vi "testGetDataTypeEvent.vi"(8 "error in (no error)":errorcluster) -> (0 "error out":errorcluster)   [LabVIEW 2018]
uses:
  src/LibReader/LibReader.lvclass
  <vilib>/addons/_JKI Toolkits/Caraya/classes/Assert/Assert Error.vi
  <vilib>/addons/_JKI Toolkits/Caraya/classes/Assert/Assert Equal Value_Variant.vi
  <vilib>/addons/_JKI Toolkits/Caraya/classes/Test/Test.lvclass
  <vilib>/addons/_JKI Toolkits/Caraya/classes/Assert/Assert.lvclass
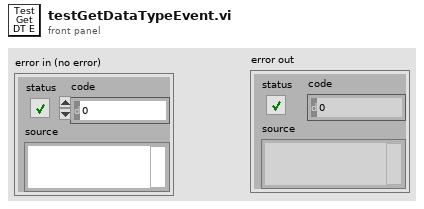
[diagram p1: front panel]
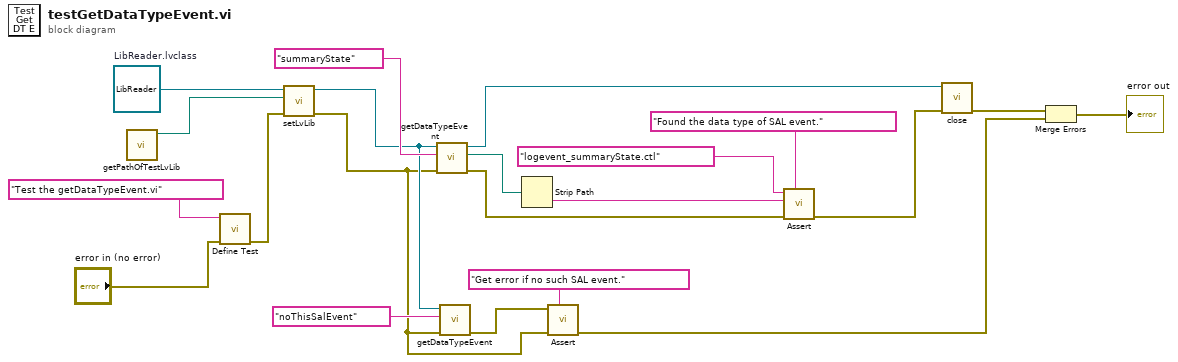
[diagram p0: block diagram]
diagram:
  w19 = refnum<class "LibReader.lvclass"> refnum  # LibReader.lvclass
  n1 = call "getPathOfTestLvLib.vi"() -> ("testLvLibPath"=w18:path)  [unwired: 11 in]
  n2 = call <vilib>:"Define Test.vi"("error in (no error)"="error in (no error)", "Label (VI Title)"="Test the getDataTypeEvent.vi") -> ("error out"=w17:errorcluster)  [unwired: 9 in]
  n3 = call "setLvLib.vi"("error in (no error)"=w17, "pathLvLib"=w18, "LibReader in"=w19) -> ("error out"=w1:errorcluster, "LibReader out"=w8:refnum<class "LibReader.lvclass">)  [unwired: 7 in]
  n4 = call "getDataTypeEvent.vi"("error in (no error)"=w1, "name"="summaryState", "LibReader in"=w8) -> ("error out"=w13:errorcluster, "pathDataType"=w15:path, "LibReader out"=w16:refnum<class "LibReader.lvclass">)  [unwired: 6 in]
  n5 = call "getDataTypeEvent.vi"("error in (no error)"=w1, "name"="noThisSalEvent", "LibReader in"=w8) -> ("error out"=w2:errorcluster)  [unwired: 6 in, 2 out]
  n6 = Strip Path(path=w15) -> (name=w14:string)  [unwired: 1 out]
  n7 = call-poly <vilib>:"Assert.vi"("Label"="Get error if no such SAL event.", "error in (no error)"=w1, "Error?"=w2) -> ("error out"=w3:errorcluster)  [unwired: 8 in]
  n8 = call-poly <vilib>:"Assert.vi"("Label"="Found the data type of SAL event.", "error in (no error)"=w13, "Y"=w14, "X"="logevent_summaryState.ctl") -> ("error out"=w12:errorcluster)  [unwired: 7 in]
  n9 = call "close.vi"("error in (no error)"=w12, "LibReader in"=w16) -> ("error out"=w5:errorcluster)  [unwired: 8 in, 1 out]
  n10 = Merge Errors(w5, w3) -> (→"error out":errorcluster)
